vi "create.vi"(8 "error in":errorcluster, 11 "parameters":T1) -> (0 "error out":errorcluster, 3 "websocket standalone server out":refnum<class "websocket standalone server.lvclass">)   [LabVIEW 2016, in "websocket standalone server.lvclass"]
uses:
  websocket standalone server.lvclass
  websocket connection parameters.ctl
  websocket sourced packet.ctl
  websocket data packet.ctl
  websocket message type.ctl
  websocket listener message.ctl
  websocket standalone server.lvclass/websocket standalone server.ctl
  listener.vi
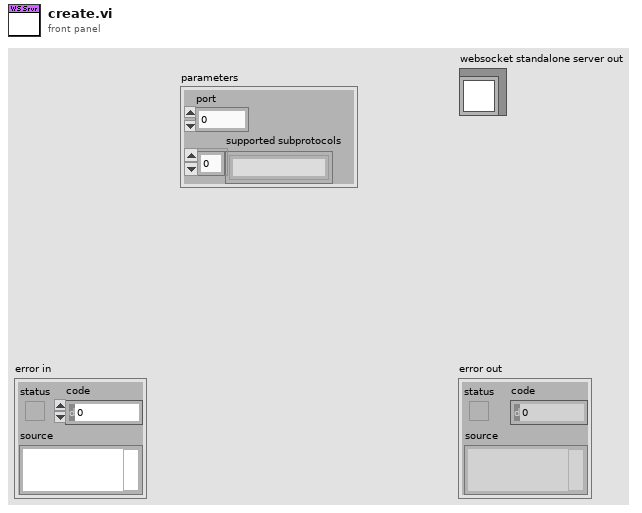
[diagram p1: front panel]
types:
  T1 = typedef "websocket standalone server.lvclass/websocket connection parameters.ctl" = cluster{"port":u16, "supported subprotocols":string[]}
  T2 = typedef "websocket standalone server.lvclass/websocket sourced packet.ctl" = cluster{"connection":refnum<queue>, "packet":T3}
  T3 = typedef "websocket standalone server.lvclass/websocket data packet.ctl" = cluster{"message type":T4, "data":string}
  T4 = typedef "websocket standalone server.lvclass/websocket message type.ctl" = enum16{"UTF8 data", "binary data", "close", "ping", "pong"}
  T5 = typedef "websocket standalone server.lvclass/websocket listener message.ctl" = enum16{"exit", "block socket", "unblock socket"}
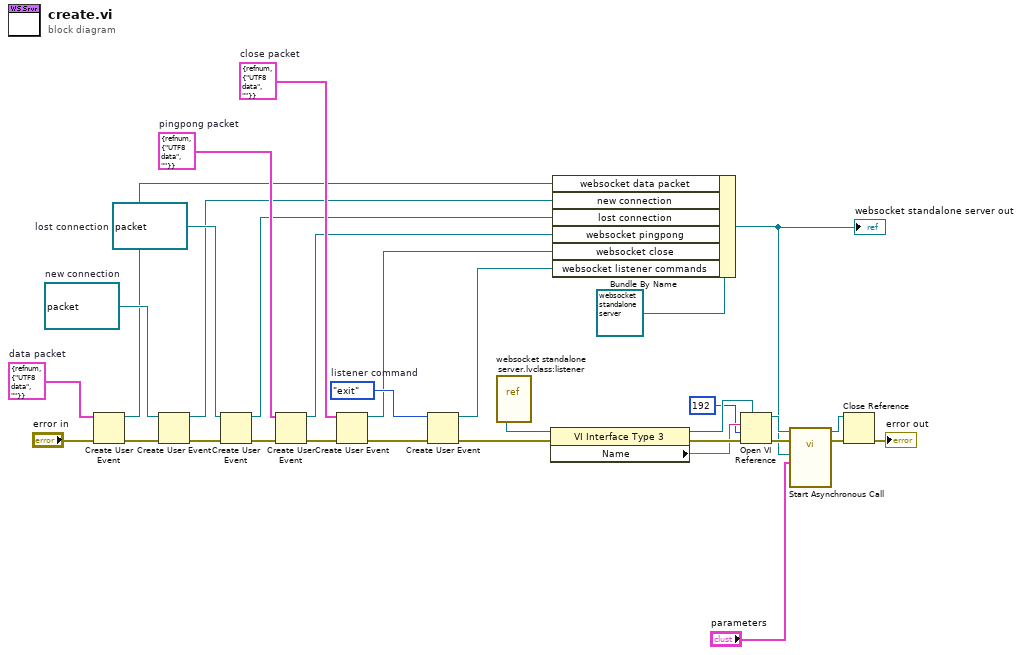
[diagram p0: block diagram]
diagram:
  w15 = T2 {"connection"=refnum, "packet"={"message type"=enum."UTF8 data", "data"=""}}  # close packet
  w14 = T2 {"connection"=refnum, "packet"={"message type"=enum."UTF8 data", "data"=""}}  # pingpong packet
  w16 = refnum<queue> refnum  # lost connection
  w17 = refnum<queue> refnum  # new connection
  w18 = websocket_listener_message."exit"  # listener command
  w20 = T2 {"connection"=refnum, "packet"={"message type"=enum."UTF8 data", "data"=""}}  # data packet
  n1 = Create User Event(user event datatype=w20, error in="error in") -> (user event=w8:refnum<user-event>, error out=w13:errorcluster)
  n2 = Create User Event(user event datatype=w17, error in=w13) -> (user event=w7:refnum<user-event>, error out=w12:errorcluster)
  n3 = Create User Event(user event datatype=w16, error in=w12) -> (user event=w6:refnum<user-event>, error out=w11:errorcluster)
  n4 = Create User Event(user event datatype=w14, error in=w11) -> (user event=w5:refnum<user-event>, error out=w10:errorcluster)
  n5 = Create User Event(user event datatype=w15, error in=w10) -> (user event=w4:refnum<user-event>, error out=w9:errorcluster)
  n6 = Create User Event(user event datatype=w18, error in=w9) -> (user event=w1:refnum<user-event>, error out=w19:errorcluster)
  n7 = vi-ref "websocket standalone server.lvclass:listener.vi"() -> (w31:refnum<vi>)
  n8 = property class="VI Interface Type 3"(reference=w31, error in=w19) -> (reference out=w27:refnum<vi>, error out=w29:errorcluster, "Name"=w28:string)
  n9 = Bundle By Name(cluster=refnum<class "websocket standalone server.lvclass"> refnum ("websocket standalone server in"), "websocket data packet"=w8, "new connection"=w7, "lost connection"=w6, "websocket pingpong"=w5, "websocket close"=w4, "websocket listener commands"=w1) -> (w2:refnum<class "websocket standalone server.lvclass">)
  "websocket standalone server out" <- w2
  n10 = Open VI Reference(type specifier VI Refnum (for type only)=w27, vi path=w28, options=192, error in (no error)=w29) -> (vi reference=w24:refnum<vi>, error out=w25:errorcluster)  [unwired: 2 in]
  n11 = call-by-ref "Start Asynchronous Call"(reference=w24, error in=w25, "parameters"="parameters", "websocket standalone server in"=w2) -> (reference out=w22:refnum<vi>, error out=w23:errorcluster)  [unwired: 10 in]
  n12 = Close Reference(reference=w22, error in (no error)=w23) -> (error out=→"error out":errorcluster)
